vi "myRIO_BRig_FPGA_v3,40__PortC__v2.vi"() -> ()   [LabVIEW 2014]
uses:
  <vilib>/rvi/FXPMathLib/FxpDiv/subVIs/nifxpmath_Div_SimConfig.ctl
  <vilib>/rvi/FXPMathLib/FxpSinAndCos/subVIs/nifxpmath_SinAndCos_SimConfig.ctl
  <vilib>/rvi/FXPMathLib/FxpDiv/simVIs/DllFxpDivTemp_sub.vi
  <vilib>/rvi/FXPMathLib/FxpSinAndCos/simVIs/DllFxpSinAndCosTemp_sub.vi
  <vilib>/rvi/Emulation/niFpgaGetClockAttributes.vi
  <vilib>/rvi/Emulation/niFpgaSctlEmulationGetInTimedLoop.vi
  <vilib>/rvi/Emulation/niFpgaEmulationReportErrorSimple.vi
  <vilib>/rvi/eio/common/nirviEmuTemplateMethod_errors.vi
  <vilib>/rvi/Emulation/niFpgaCriticalErrorInLSC.vi
  <vilib>/rvi/FXPMathLib/FxpDiv/XNode/nifxpmath_Div.xnode
  <vilib>/rvi/FXPMathLib/FxpMul/XNode/nifxpmath_Multiplier.xnode
  <vilib>/rvi/FXPMathLib/FxpSinAndCos/XNode/nifxpmath_SinAndCos.xnode
  <vilib>/rvi/FXPMathLib/FxpSub/XNode/nifxpmath_Sub.xnode
  <vilib>/eio/EIONode/EIONode.xnode
  <vilib>/rvi/FXPMathLib/sim/FxpSim.dll
panel:
  in  "laser_Nshutter":u32=100
  in  "AnaOut_0":i16
  in  "f_time_select":u32=173
  in  "laser_Nvalley":u32=100
  in  "laser_Npeak":u32=100
  in  "laserledMTrig":bool
  in  "tCycle_laser_wro":u32=100
  in  "tDelay_laser_wro":u32
  in  "tCycle_laser_rew":u32=100
  in  "tDelay_laser_rew":u32
  in  "laserResponse_reward_LED":bool
  in  "laserResponse_wrong_LED":bool
  out "SelectWrong":bool
  out "SelectReward":bool
  in  "laserResponse_wrong":bool
  in  "laserResponse_reward":bool
  in  "Left(F)_or_Right(T)":bool
  in  "ignoreWrong":bool
  in  "SelectionState":bool
  in  "laserMTrig":bool
  in  "FPGA_Stop":bool
  in  "audioTrigger_L":bool
  in  "audioTrigger_R":bool
  in  "audioFreq_L_Hz":u16=1000 min=1000 max=14000 step=1000
  in  "audioAmp_L":u16=1 min=1 max=32767 step=1
  in  "audioFreq_R_Hz":u16=1000 min=1000 max=14000 step=1000
  in  "audioAmp_R":u16=1 min=1 max=32767 step=1
  in  "A3_SL":bool
  in  "A1_SR":bool
  in  "Counts_Reset":bool
  out "A4_LickR":u32
  out "A2_LickL":u32
  in  "A6_Act":bool
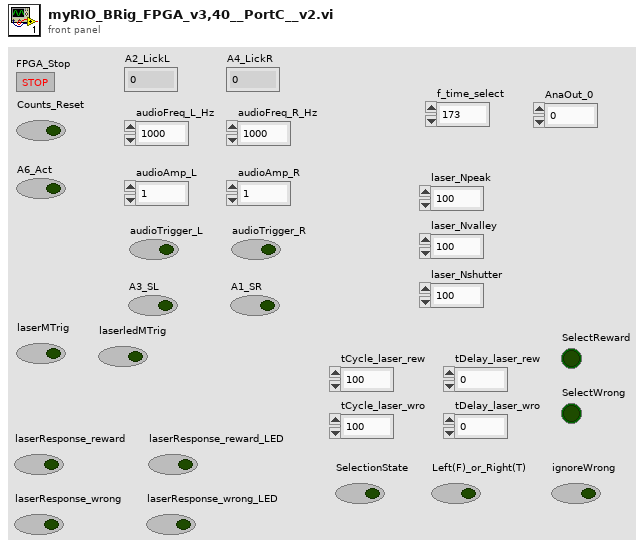
[diagram p1: front panel]
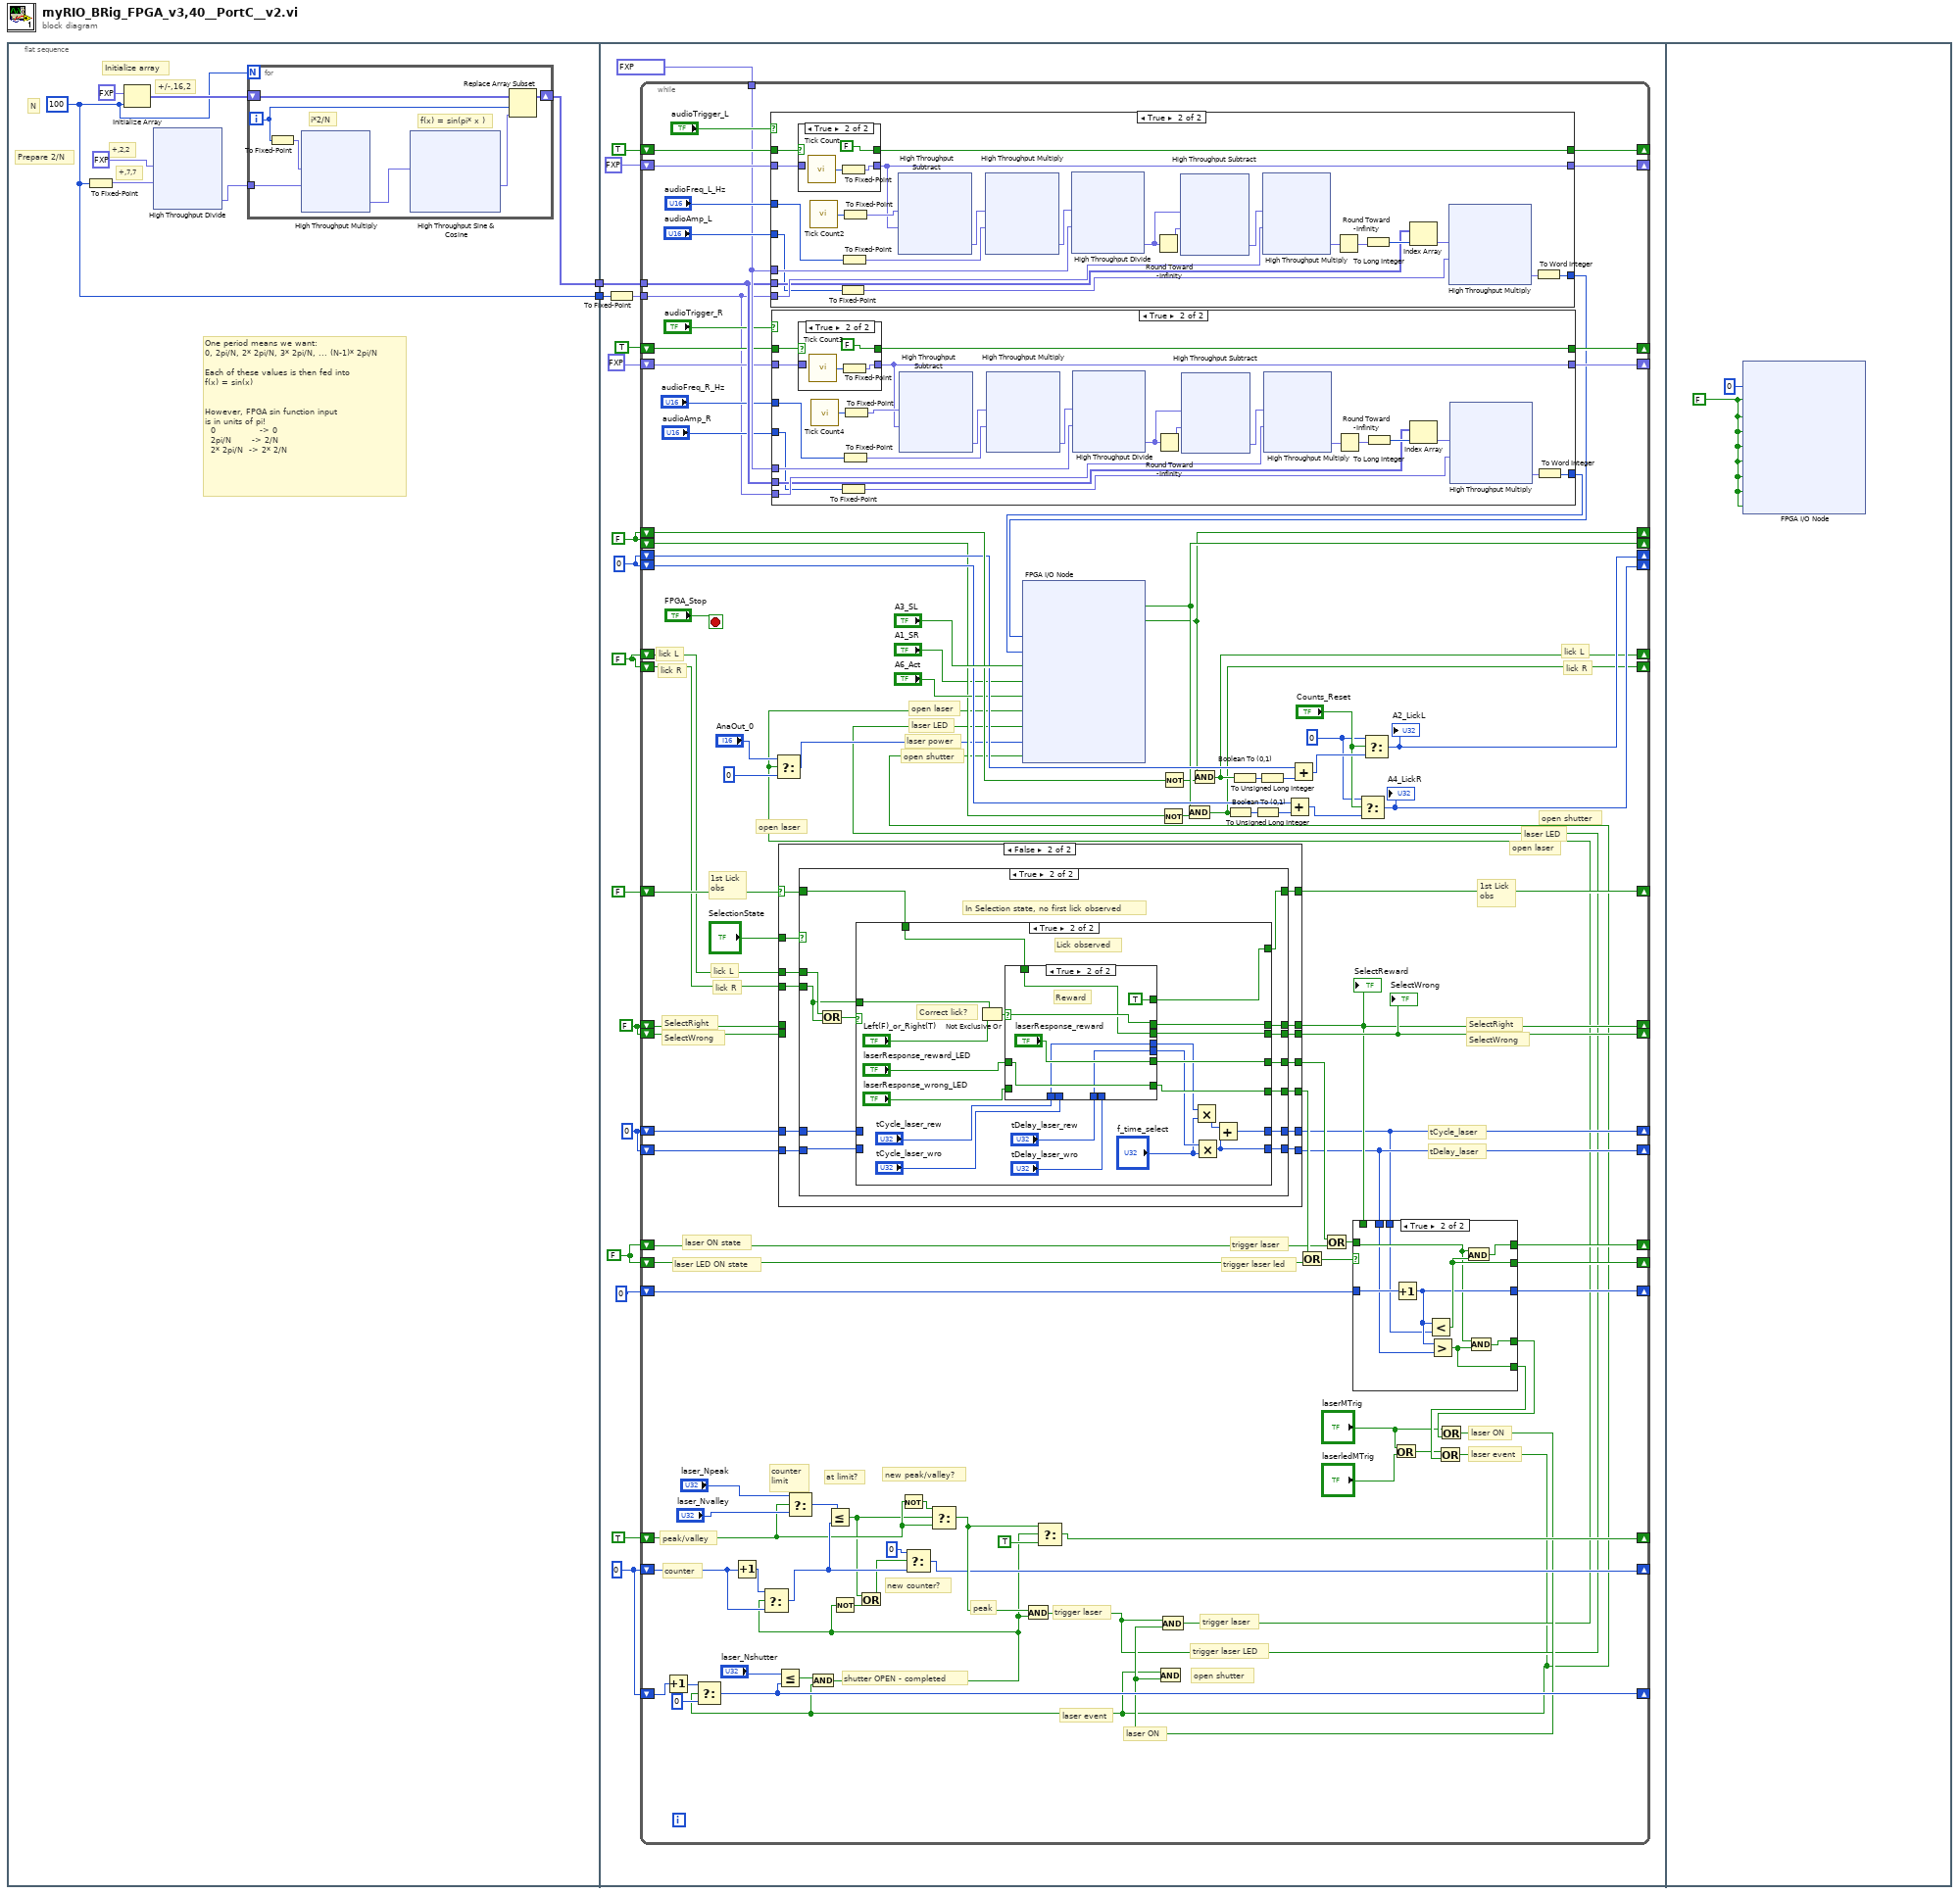
[diagram p0: block diagram]
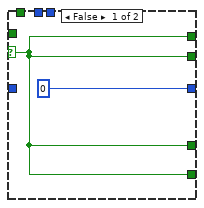
[diagram p2: hidden frame]
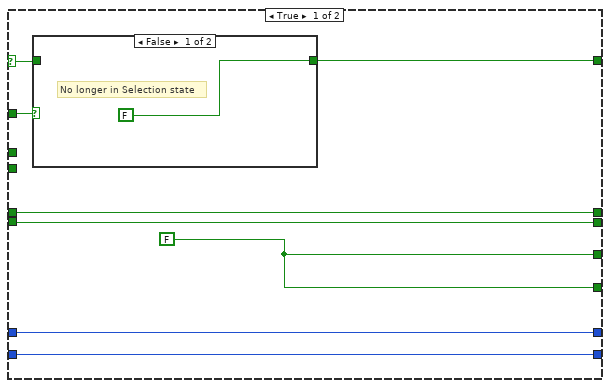
[diagram p3: hidden frame]
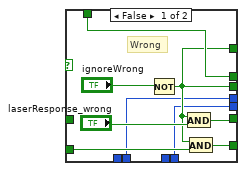
[diagram p7: hidden frame]
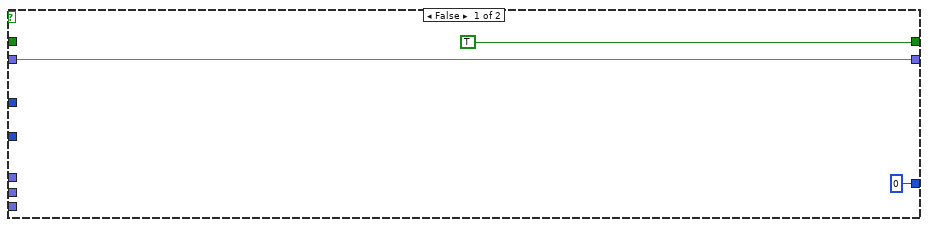
[diagram p8: hidden frame]
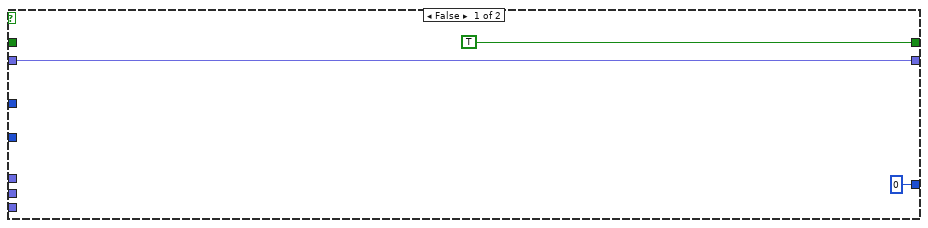
[diagram p10: hidden frame]
diagram:
  n1 = flat-sequence {
    tunnel: [w4] -> w2
    tunnel: [w3] -> w1
    tunnel: w2 -> [w86]
    tunnel: w1 -> [w88]
    frame #0 {
      w3 = 100 ("dimension size")
      # "N"
      # "+,7,7"
      # "+,2,2"
      # "+/-,16,2"
      # "Prepare 2/N"
      # "One period means we want:\n0, 2pi/N, 2* 2pi/N, 3* 2pi/N, ... (N-1)* 2pi/N\n\nEach of these values is then fed into\nf(x) = sin(x)\n\n\nHowever, FPGA sin function input\nis in units of pi!\n  0               -> 0\n  2pi/N       -> 2/N\n  2* 2pi/N  -> 2* 2/N"
      # "Initialize array"
      n2 = To Fixed-Point(number=w3) -> (fixed-point=w6:fxp<+,7,7>)  [unwired: 1 in]
      n3 = Initialize Array(fxp<+/-,16,2> 0.0 ("element"), w3) -> (w9:fxp<+/-,16,2>[])
      n4 = xnode "High Throughput Divide"("x"=fxp<+,2,2> 2.0, "y"=w6) -> ("x/y"=w5:fxp<+,27,0>)
      n5 = for {
        N: w3 -> [_]
        shift-right: [w42] -> w4
        shift-left: w9 -> [w43]
        tunnel: w5 -> [w38]
        i -> [w41]
        # "f(x) = sin(pi* x )"
        # "i*2/N"
        n6 = To Fixed-Point(number=w41) -> (fixed-point=w39:fxp<+,7,7>)  [unwired: 1 in]
        n7 = xnode ("High Throughput Multiply")("x"=w39, "y"=w38) -> ("x*y"=w37:fxp<+,34,7>)
        n8 = xnode "High Throughput Sine & Cosine"("x (pi)"=w37) -> ("sin(x)"=w40:fxp<+/-,16,2>)  [unwired: 1 out]
        n9 = Replace Array Subset(array=w43, new element=w40, index=w41) -> (w42:fxp<+/-,16,2>[])
      }
    }
    frame #1 {
      w74 = u32 0
      w76 = u32 0
      w78 = FALSE
      w77 = FALSE
      w81 = FALSE
      w82 = FALSE
      w83 = u32 0
      n10 = To Fixed-Point(number=w88) -> (fixed-point=w87:fxp<+,7,7>)  [unwired: 1 in]
      n11 = while {
        shift-right: [w186] -> _
        shift-left: TRUE -> [w190]
        shift-right: [w185] -> _
        shift-left: fxp<+,32,32> 0.0 -> [w189]
        tunnel: fxp<+,17,26> 40000000.0 -> [w184]
        tunnel: w87 -> [w177]
        tunnel: w86 -> [w183]
        shift-right: [w176] -> _
        shift-left: TRUE -> [w182]
        shift-right: [w175] -> _
        shift-left: fxp<+,32,32> 0.0 -> [w181]
        shift-right: [w153] -> _
        shift-left: w83 -> [w165]
        shift-right: [w156] -> _
        shift-left: w83 -> [w169]
        shift-right: [w157] -> _
        shift-left: w82 -> [w160]
        shift-right: [w154] -> _
        shift-left: w82 -> [w166]
        shift-right: [w151] -> _
        shift-left: FALSE -> [w150]
        shift-right: [w149] -> _
        shift-left: w81 -> [w147]
        shift-right: [w148] -> _
        shift-left: w81 -> [w146]
        shift-right: [w136] -> _
        shift-left: w77 -> [w138]
        shift-right: [w144] -> _
        shift-left: u32 0 -> [w145]
        shift-right: [w130] -> _
        shift-left: w78 -> [w142]
        shift-right: [w143] -> _
        shift-left: w78 -> [w141]
        shift-right: [w137] -> _
        shift-left: w77 -> [w134]
        shift-right: [w126] -> _
        shift-left: w76 -> [w129]
        shift-right: [w127] -> _
        shift-left: w76 -> [w128]
        shift-right: [w110] -> _
        shift-left: w74 -> [w120]
        shift-right: [w111] -> _
        shift-left: TRUE -> [w114]
        shift-right: [w99] -> _
        shift-left: w74 -> [w103]
        stop <- "FPGA_Stop" stop-if-true
        w162 = u32 0
        # "open shutter"
        # "laser LED"
        # "open laser"
        # "open laser"
        # "trigger laser LED"
        # "trigger laser"
        # "open shutter"
        # "laser ON"
        # "laser power"
        # "open laser"
        # "laser LED"
        # "open shutter"
        # "shutter OPEN - completed"
        # "trigger laser"
        # "peak"
        # "laser event"
        # "new peak/valley?"
        # "counter"
        # "peak/valley"
        # "new counter?"
        # "at limit?"
        # "counter\nlimit"
        # "tDelay_laser"
        # "tCycle_laser"
        # "laser event"
        # "laser ON"
        # "laser LED ON state"
        # "laser ON state"
        # "SelectWrong"
        # "SelectRight"
        # "SelectWrong"
        # "SelectRight"
        # "lick R"
        # "lick L"
        # "1st Lick\nobs"
        # "1st Lick\nobs"
        # "lick R"
        # "lick L"
        # "lick R"
        # "lick L"
        # "trigger laser led"
        # "trigger laser"
        n12 = Increment(x=w103) -> (x+1=w102:u32)
        n13 = Increment(x=w120) -> (x+1=w119:u32)
        n14 = case shown="True" "audioTrigger_L" {
          tunnel: w190 -> [_ w368]
          tunnel: w189 -> [w344 w367]
          tunnel: "audioFreq_L_Hz" -> [_ w364]
          tunnel: w184 -> [_ w361]
          tunnel: [w344 w345] -> w185
          tunnel: [TRUE w358] -> w186
          tunnel: w177 -> [_ w357]
          tunnel: w183 -> [_ w352]
          tunnel: "audioAmp_L" -> [_ w350]
          tunnel: [i16 0 w347] -> w172
          frame False {
          }
          frame True {
            n15 = case shown="True" w368 {
              selector: w368 -> [w397 _]
              tunnel: [w397 FALSE] -> w358
              tunnel: w367 -> [w396 _]
              tunnel: [w396 w398] -> w345
              frame False {
              }
              frame True {
                n16 = call "Tick Count"() -> ("Tick Count(Ticks)"=w400:u32)
                n17 = To Fixed-Point(number=w400) -> (fixed-point=w398:fxp<+,32,32>)  [unwired: 1 in]
              }
            }
            n18 = call "Tick Count2"() -> ("Tick Count(Ticks)"=w366:u32)
            n19 = To Fixed-Point(number=w350) -> (fixed-point=w349:fxp<+,15,15>)  [unwired: 1 in]
            n20 = To Fixed-Point(number=w364) -> (fixed-point=w363:fxp<+,14,14>)  [unwired: 1 in]
            n21 = To Fixed-Point(number=w366) -> (fixed-point=w346:fxp<+,32,32>)  [unwired: 1 in]
            n22 = xnode "High Throughput Subtract"("x"=w346, "y"=w345) -> ("x-y"=w365:fxp<+,32,32>)
            n23 = xnode ("High Throughput Multiply")("x"=w365, "y"=w363) -> ("x*y"=w362:fxp<+,46,46>)
            n24 = xnode "High Throughput Divide"("x"=w362, "y"=w361) -> ("x/y"=w360:fxp<+,34,21>)
            n25 = Round Toward -Infinity(1:w360) -> (0:w359:fxp<+,21,21>)
            n26 = xnode "High Throughput Subtract"("x"=w360, "y"=w359) -> ("x-y"=w356:fxp<+,14,1>)
            n27 = xnode ("High Throughput Multiply")("x"=w356, "y"=w357) -> ("x*y"=w353:fxp<+,21,8>)
            n28 = Round Toward -Infinity(1:w353) -> (0:w355:fxp<+,8,8>)
            n29 = To Long Integer(number=w355) -> (32bit integer=w354:i32)
            n30 = Index Array(array=w352, index=w354) -> (element=w351:fxp<+/-,16,2>)
            n31 = xnode ("High Throughput Multiply")("x"=w351, "y"=w349) -> ("x*y"=w348:fxp<+/-,31,17>)
            n32 = To Word Integer(number=w348) -> (16bit integer=w347:i16)
          }
        }
        n33 = case shown="True" "audioTrigger_R" {
          tunnel: w182 -> [_ w309]
          tunnel: w181 -> [w285 w308]
          tunnel: "audioFreq_R_Hz" -> [_ w305]
          tunnel: w184 -> [_ w302]
          tunnel: [w285 w286] -> w175
          tunnel: [TRUE w299] -> w176
          tunnel: w177 -> [_ w298]
          tunnel: w183 -> [_ w293]
          tunnel: "audioAmp_R" -> [_ w291]
          tunnel: [i16 0 w288] -> w173
          frame False {
          }
          frame True {
            n34 = case shown="True" w309 {
              selector: w309 -> [w338 _]
              tunnel: [w338 FALSE] -> w299
              tunnel: w308 -> [w337 _]
              tunnel: [w337 w339] -> w286
              frame False {
              }
              frame True {
                n35 = call "Tick Count3"() -> ("Tick Count(Ticks)"=w341:u32)
                n36 = To Fixed-Point(number=w341) -> (fixed-point=w339:fxp<+,32,32>)  [unwired: 1 in]
              }
            }
            n37 = call "Tick Count4"() -> ("Tick Count(Ticks)"=w307:u32)
            n38 = To Fixed-Point(number=w291) -> (fixed-point=w290:fxp<+,15,15>)  [unwired: 1 in]
            n39 = To Fixed-Point(number=w305) -> (fixed-point=w304:fxp<+,14,14>)  [unwired: 1 in]
            n40 = To Fixed-Point(number=w307) -> (fixed-point=w287:fxp<+,32,32>)  [unwired: 1 in]
            n41 = xnode "High Throughput Subtract"("x"=w287, "y"=w286) -> ("x-y"=w306:fxp<+,32,32>)
            n42 = xnode ("High Throughput Multiply")("x"=w306, "y"=w304) -> ("x*y"=w303:fxp<+,46,46>)
            n43 = xnode "High Throughput Divide"("x"=w303, "y"=w302) -> ("x/y"=w301:fxp<+,34,21>)
            n44 = Round Toward -Infinity(1:w301) -> (0:w300:fxp<+,21,21>)
            n45 = xnode "High Throughput Subtract"("x"=w301, "y"=w300) -> ("x-y"=w297:fxp<+,14,1>)
            n46 = xnode ("High Throughput Multiply")("x"=w297, "y"=w298) -> ("x*y"=w294:fxp<+,21,8>)
            n47 = Round Toward -Infinity(1:w294) -> (0:w296:fxp<+,8,8>)
            n48 = To Long Integer(number=w296) -> (32bit integer=w295:i32)
            n49 = Index Array(array=w293, index=w295) -> (element=w292:fxp<+/-,16,2>)
            n50 = xnode ("High Throughput Multiply")("x"=w292, "y"=w290) -> ("x*y"=w289:fxp<+/-,31,17>)
            n51 = To Word Integer(number=w289) -> (16bit integer=w288:i16)
          }
        }
        n52 = case shown="False" w150 {
          selector: w150 -> [w209 w224]
          tunnel: "SelectionState" -> [w211 w226]
          tunnel: [w210 w225] -> w151
          tunnel: w147 -> [_ w223]
          tunnel: w146 -> [_ w222]
          tunnel: [w208 w221] -> w135
          tunnel: [w206 w220] -> w130
          tunnel: [w207 w219] -> w143
          tunnel: w142 -> [w206 _]
          tunnel: w141 -> [w207 _]
          tunnel: [w208 w218] -> w139
          tunnel: [w205 w217] -> w126
          tunnel: [w204 w216] -> w127
          tunnel: w129 -> [w205 w215]
          tunnel: w128 -> [w204 w214]
          frame True {
            w208 = FALSE
            n53 = case shown="False" w211 {
              tunnel: [FALSE w213] -> w210
              tunnel: w209 -> [_ w213]
              frame False {
                # "No longer in Selection state"
              }
              frame True {
                # "Already observed first lick, no other action"
              }
            }
          }
          frame False {
            n54 = case shown="True" w226 {
              tunnel: [w229 w239] -> w225
              tunnel: w224 -> [w229 w235]
              tunnel: w223 -> [_ w241]
              tunnel: w222 -> [_ w240]
              tunnel: [w229 w238] -> w221
              tunnel: [w229 w237] -> w220
              tunnel: [w229 w236] -> w219
              tunnel: [w229 w234] -> w218
              tunnel: [w228 w233] -> w217
              tunnel: [w227 w232] -> w216
              tunnel: w215 -> [w228 w231]
              tunnel: w214 -> [w227 w230]
              frame False {
                # "Not in Selection state"
              }
              frame True {
                # "In Selection state, no first lick observed"
                n55 = Or(x=w241, y=w240) -> (x .or. y?=w242:bool)
                n56 = case shown="True" w242 {
                  tunnel: w240 -> [_ w265]
                  tunnel: [w245 w258] -> w239
                  tunnel: [w245 w263] -> w238
                  tunnel: [w245 w262] -> w237
                  tunnel: [w245 w261] -> w236
                  tunnel: w235 -> [w245 w260]
                  tunnel: [w245 w259] -> w234
                  tunnel: [w244 w247] -> w233
                  tunnel: [w243 w246] -> w232
                  tunnel: w231 -> [w244 _]
                  tunnel: w230 -> [w243 _]
                  frame False {
                  }
                  frame True {
                    # "Correct lick?"
                    # "Lick observed"
                    n57 = Not Exclusive Or(1:"Left(F)_or_Right(T)", 2:w265) -> (0:w264:bool)
                    n58 = case shown="True" w264 {
                      selector: w264 -> [_ w281]
                      tunnel: [w272 "laserResponse_reward"] -> w263
                      tunnel: [w270 w277] -> w261
                      tunnel: [w274 w281] -> w262
                      tunnel: w260 -> [w274 w277]
                      tunnel: [w271 w279] -> w259
                      tunnel: [w270 TRUE] -> w258
                      tunnel: "laserResponse_reward_LED" -> [_ w279]
                      tunnel: "laserResponse_wrong_LED" -> [w269 _]
                      tunnel: "tCycle_laser_rew" -> [_ w276]
                      tunnel: "tCycle_laser_wro" -> [w267 _]
                      tunnel: "tDelay_laser_rew" -> [_ w278]
                      tunnel: "tDelay_laser_wro" -> [w268 _]
                      tunnel: [w268 w278] -> w250
                      tunnel: [w267 w276] -> w249
                      frame False {
                        # "Wrong"
                        n59 = Not(x="ignoreWrong") -> (.not. x?=w270:bool)
                        n60 = And(x=w270, y="laserResponse_wrong") -> (x .and. y?=w272:bool)
                        n61 = And(x=w270, y=w269) -> (x .and. y?=w271:bool)
                      }
                      frame True {
                        # "Reward"
                      }
                    }
                    n62 = Multiply(x=w249, y="f_time_select") -> (x*y=w251:u32)
                    n63 = Multiply(x=w250, y="f_time_select") -> (x*y=w246:u32)
                    n64 = Add(x=w251, y=w246) -> (x+y=w247:u32)
                  }
                }
              }
            }
          }
        }
        "SelectWrong" <- w143
        "SelectReward" <- w130
        n65 = Select(t="laser_Npeak", s=w114, f="laser_Nvalley") -> (s? t:f=w122:u32)
        n66 = Not(x=w114) -> (.not. x?=w115:bool)
        n67 = Not(x=w160) -> (.not. x?=w159:bool)
        n68 = Not(x=w166) -> (.not. x?=w155:bool)
        n69 = Or(x=w139, y=w138) -> (x .or. y?=w140:bool)
        n70 = Or(x=w135, y=w134) -> (x .or. y?=w133:bool)
        n71 = case shown="True" w140 {
          selector: w140 -> [w193 _]
          tunnel: w145 -> [_ w203]
          tunnel: [u32 0 w200] -> w144
          tunnel: [w193 w201] -> w136
          tunnel: [w193 w202] -> w137
          tunnel: w133 -> [_ w199]
          tunnel: [w193 w198] -> w131
          tunnel: [w193 w197] -> w132
          tunnel: w130 -> [_ _]
          tunnel: w127 -> [_ w196]
          tunnel: w126 -> [_ w195]
          frame False {
          }
          frame True {
            n72 = Increment(x=w203) -> (x+1=w200:u32)
            n73 = Less?(x=w200, y=w195) -> (x < y?=w201:bool)
            n74 = Greater?(x=w200, y=w196) -> (0:w198:bool)
            n75 = And(x=w199, y=w201) -> (x .and. y?=w202:bool)
            n76 = And(x=w199, y=w198) -> (x .and. y?=w197:bool)
          }
        }
        n77 = Or(x="laserMTrig", y="laserledMTrig") -> (x .or. y?=w124:bool)
        n78 = Or(x=w124, y=w131) -> (x .or. y?=w92:bool)
        n79 = Select(t=w102, s=w92, f=u32 0) -> (s? t:f=w99:u32)
        n80 = Less Or Equal?(x="laser_Nshutter", y=w99) -> (x <= y?=w98:bool)
        n81 = And(x=w98, y=w92) -> (x .and. y?=w96:bool)
        n82 = Select(t=w119, s=w96, f=w120) -> (s? t:f=w118:u32)
        n83 = Less Or Equal?(x=w122, y=w118) -> (x <= y?=w108:bool)
        n84 = Not(x=w96) -> (.not. x?=w109:bool)
        n85 = Or(x=w108, y=w109) -> (x .or. y?=w107:bool)
        n86 = Select(t=u32 0, s=w107, f=w118) -> (s? t:f=w110:u32)
        n87 = Select(t=w115, s=w108, f=w114) -> (s? t:f=w113:bool)
        n88 = And(x=w113, y=w96) -> (x .and. y?=w93:bool)
        n89 = Select(t=w113, s=w96, f=TRUE) -> (s? t:f=w111:bool)
        n90 = Or(x="laserMTrig", y=w132) -> (x .or. y?=w95:bool)
        n91 = And(x=w92, y=w95) -> ()  [unwired: 1 out]
        n92 = And(x=w93, y=w95) -> (x .and. y?=w94:bool)
        n93 = Select(t="AnaOut_0", s=w94, f=i16 0) -> (s? t:f=w106:i16)
        n94 = xnode "FPGA I/O Node"("AudioOut/Left"=w172, "AudioOut/Right"=w173, "ConnectorC/DIO3"="A3_SL", "ConnectorC/DIO1"="A1_SR", "ConnectorC/DIO7"="A6_Act", "ConnectorC/DIO0"=w94, "ConnectorC/DIO5"=w93, "ConnectorC/AO0"=w106, "ConnectorC/DIO6"=w92) -> ("ConnectorC/DIO4"=w157:bool, "ConnectorC/DIO2"=w154:bool)  [unwired: 11 in, 11 out]
        n95 = And(x=w157, y=w159) -> (x .and. y?=w148:bool)
        n96 = And(x=w154, y=w155) -> (x .and. y?=w149:bool)
        n97 = Boolean To (0,1)(Boolean=w148) -> (0, 1=w171:i16)
        n98 = Boolean To (0,1)(Boolean=w149) -> (0, 1=w168:i16)
        n99 = To Unsigned Long Integer(number=w171) -> (unsigned 32bit integer=w170:u32)
        n100 = To Unsigned Long Integer(number=w168) -> (unsigned 32bit integer=w167:u32)
        n101 = Add(x=w169, y=w170) -> (x+y=w158:u32)
        n102 = Add(x=w165, y=w167) -> (x+y=w164:u32)
        n103 = Select(t=w162, s="Counts_Reset", f=w158) -> (s? t:f=w156:u32)
        "A4_LickR" <- w156
        n104 = Select(t=w162, s="Counts_Reset", f=w164) -> (s? t:f=w153:u32)
        "A2_LickL" <- w153
      }
    }
    frame #2 {
      w401 = FALSE ("ConnectorA/DIO3")
      n105 = xnode "FPGA I/O Node"("ConnectorC/AO0"=i16 0 ("ConnectorA/AO0"), "ConnectorC/DIO0"=w401, "ConnectorC/DIO1"=w401, "ConnectorC/DIO2"=w401, "ConnectorC/DIO3"=w401, "ConnectorC/DIO4"=w401, "ConnectorC/DIO5"=w401, "ConnectorC/DIO6"=w401, "ConnectorC/DIO7"=w401) -> ()  [unwired: 9 in, 9 out]
    }
  }
